vi "Send GetRecord.vi"(7 "Message Priority (Normal)":T2=enum."Normal", 8 "error in (no error)":errorcluster, 10 "Label":string, 11 "Message Enqueuer":refnum<class "Message Enqueuer.lvclass">) -> (0 "error out":errorcluster, 2 "RecordData":T1 {"StopTime" format="%<%x %.3X>T"; "StartTime" format="%<%x %.3X>T"}, 3 "Message Enqueuer out":refnum<class "Message Enqueuer.lvclass">)   [LabVIEW 2025, in "Task_Abstr.lvlib" / "GetRecord Msg.lvclass"]
doc: "This VI sends the message to an actor."
uses:
  GetRecord Msg.lvclass
  <vilib>/ActorFramework/Message Enqueuer/Message Enqueuer.lvclass
  <vilib>/ActorFramework/Message Enqueuer/Message Priority.ctl
  C:/Program Files (x86)/National Instruments/LabVIEW 2025/vi.lib/ActorFramework/Message/Message.lvclass
  GetRecord Msg.lvclass/GetRecord Msg.ctl
  <vilib>/ActorFramework/Message Enqueuer/Message Enqueuer.lvclass/Message Enqueuer.ctl
  <vilib>/ActorFramework/Message Priority Queue/Priority Enqueue.vi
  D:/Hardware/DAQ/DAQ_Abstr/Task_Abstr/Task_Abstr Messages/GetRecord Msg/GetRecord Msg.lvclass
  Task_Abstr/WaveformData.ctl
  Task_Abstr/Task_Abstr.lvclass
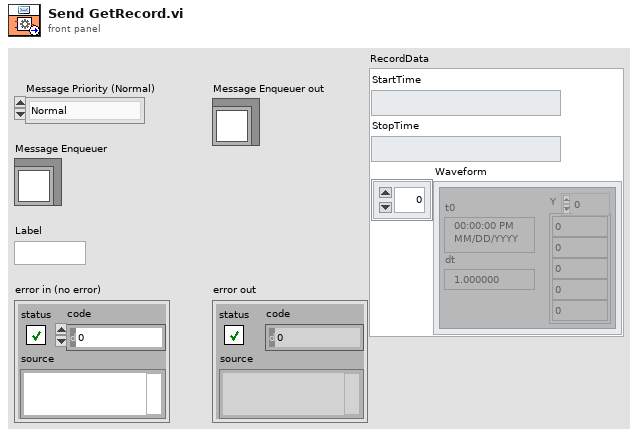
[diagram p1: front panel]
types:
  T1 = typedef "Task_Abstr.lvlib/Task_Abstr.lvclass/WaveformData.ctl" = cluster{"StartTime":timestamp, "StopTime":timestamp, "Waveform":waveform(dbl)[]}
  T2 = typedef "Actor Framework.lvlib/Message Enqueuer.lvclass/Message Priority.ctl" = enum16{"Low", "Normal", "High"}
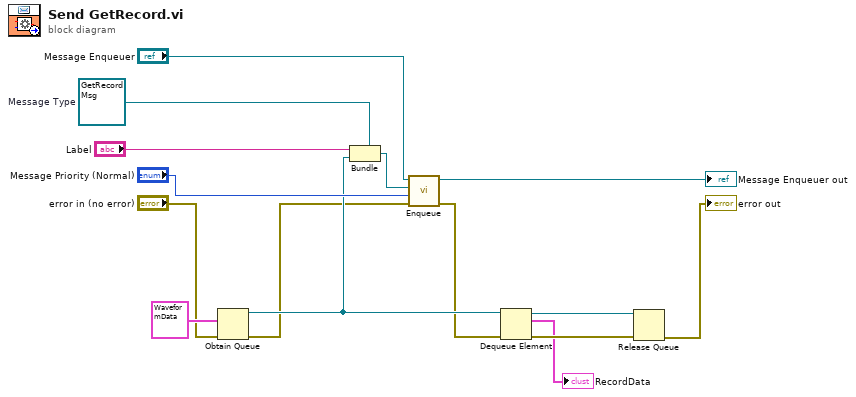
[diagram p0: block diagram]
diagram:
  w14 = refnum<class "GetRecord Msg.lvclass"> refnum  # Message Type
  n1 = Obtain Queue(element data type=T1 {"StartTime"=timestamp(0 s since 1904-01-01), "StopTime"=timestamp(0 s since 1904-01-01), "Waveform"=[]} ("WaveformData"), error in (no error)="error in (no error)") -> (queue out=w8:refnum<queue>, error out=w5:errorcluster)  [unwired: 3 in, 1 out]
  n2 = Bundle(cluster=w14, "Label", w8) -> (w13:refnum<class "GetRecord Msg.lvclass">)
  n3 = call <vilib>:"Enqueue.vi"("error in (no error)"=w5, "Message Priority (Normal)"="Message Priority (Normal)", "Message"=w13, "Message Enqueuer in"="Message Enqueuer") -> ("error out"=w7:errorcluster, "Message Enqueuer out"=→"Message Enqueuer out":refnum<class "Message Enqueuer.lvclass">)  [unwired: 6 in]
  n4 = Dequeue Element(queue=w8, error in (no error)=w7) -> (queue out=w4:refnum<queue>, element=→"RecordData":T1, error out=w3:errorcluster)  [unwired: 1 in, 1 out]
  n5 = Release Queue(queue=w4, error in (no error)=w3) -> (error out=→"error out":errorcluster)  [unwired: 1 in, 2 out]
